vi "Close JSON DAO.vi"(8 "error in (no error)":errorcluster, 11 "Customer DAO JSON in":refnum<class "Object DAO JSON.lvclass">) -> (0 "error out":errorcluster)   [LabVIEW 2020, in "Object DAO JSON.lvclass"]
uses:
  Object DAO JSON.lvclass
  Object DAO JSON.lvclass/Object DAO JSON.ctl
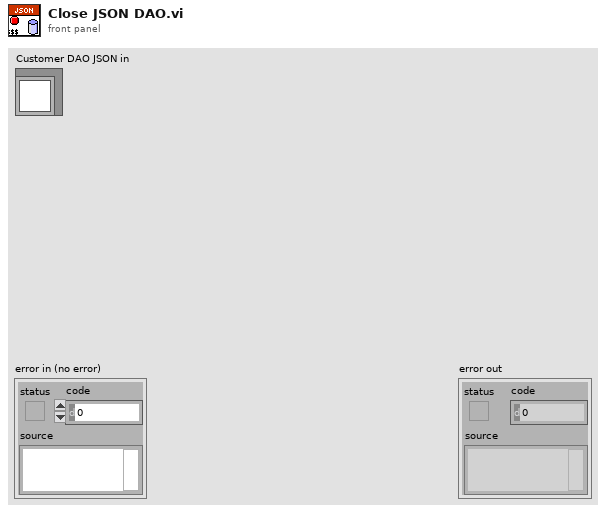
[diagram p1: front panel]
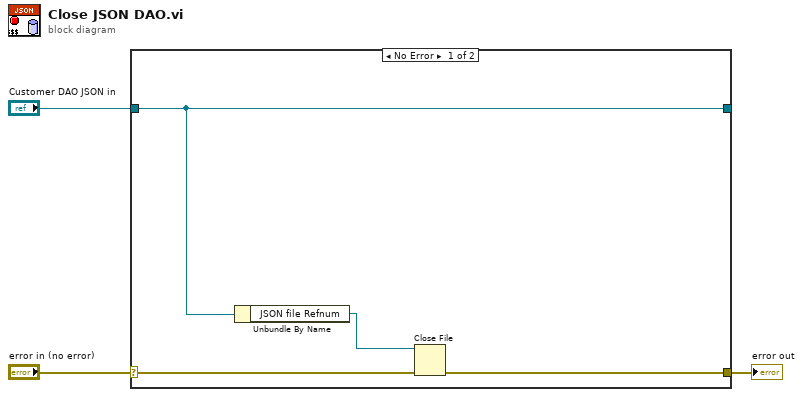
[diagram p0: block diagram]
diagram:
  n1 = case shown="No Error" "error in (no error)" {
    selector: "error in (no error)" -> [w7 w9]
    tunnel: [w6 w9] -> w2
    tunnel: [w5 w8] -> _
    tunnel: "Customer DAO JSON in" -> [w5 w8]
    frame No Error {
      n2 = Unbundle By Name(w5) -> ("JSON file Refnum"=w4:refnum<file>)
      n3 = Close File(refnum=w4, error in=w7) -> (error out=w6:errorcluster)  [unwired: 1 out]
    }
    frame Error {
    }
  }
  "error out" <- w2
